vi "produceTimingTicks.vi"(8 "error in (no error)":errorcluster, 10 "Channel":refnum<class "Channel.lvclass">, 11 "PlayFile in":refnum<class "PlayFile.lvclass">) -> (0 "error out":errorcluster, 2 "timingTick":refnum<class "ScriptEventList.lvclass">, 3 "PlayFile out":refnum<class "PlayFile.lvclass">)   [LabVIEW 2011, in "Tools.lvlib" / "Scripting.lvlib" / "PlayFile.lvclass"]
uses:
  PlayFile.lvclass
  DatabaseHelpers/Database Objects/Channel/Channel.lvclass
  ScriptEventList/ScriptEventList.lvclass
  ScriptEvent.lvclass
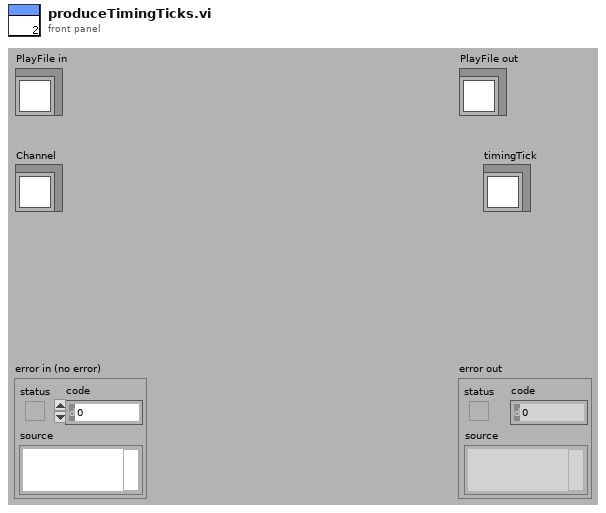
[diagram p1: front panel]
types:
  T1 = enum16{"changeValue", "pulse", "clock", "rampUp", "rampDown", "singleTone", "singleToneRamp", "playFile", "rf", "rfRamp"}
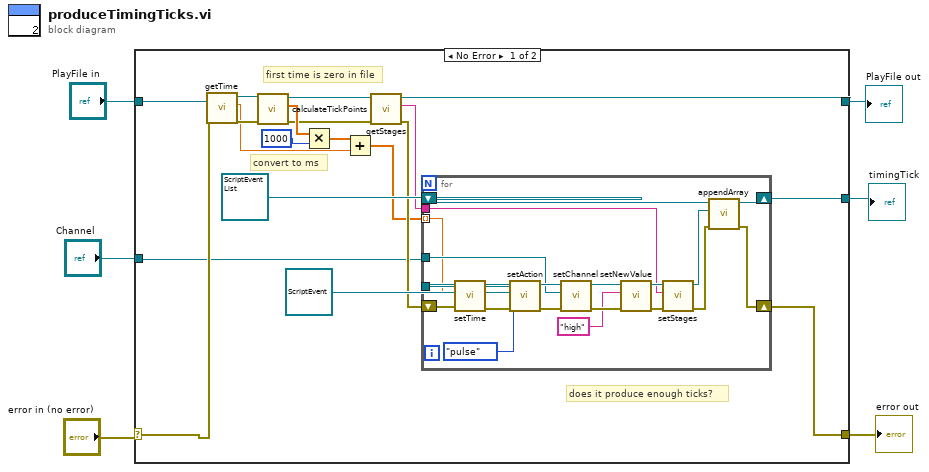
[diagram p0: block diagram]
diagram:
  n1 = case shown="No Error" "error in (no error)" {
    selector: "error in (no error)" -> [w19 w46]
    tunnel: [w20 w47] -> w5
    tunnel: "PlayFile in" -> [w21 w47]
    tunnel: [w7 w46] -> w3
    tunnel: "Channel" -> [w18 _]
    tunnel: [w8 _] -> w1
    frame No Error {
      # "convert to ms"
      # "first time is zero in file"
      # "does it produce enough ticks?"
      n2 = call "getTime.vi"("error in (no error)"=w19, "ScriptEvent.lvclass in"=w21) -> ("error out"=w16:errorcluster, "time"=w15:dbl, "ScriptEvent.lvclass out"=w17:refnum<class "PlayFile.lvclass">)  [unwired: 7 in]
      n3 = call "calculateTickPoints.vi"("error in (no error)"=w16, "PlayFile in"=w17) -> ("error out"=w9:errorcluster, "TimeArray"=w13:dbl[], "PlayFile out"=w10:refnum<class "PlayFile.lvclass">)  [unwired: 7 in]
      n4 = Multiply(x=w13, y=1000) -> (x*y=w14:dbl[])
      n5 = Add(x=w14, y=w15) -> (x+y=w11:dbl[])
      n6 = call "getStages.vi"("error in (no error)"=w9, "ScriptEvent.lvclass in"=w10) -> ("error out"=w23:errorcluster, "Stage"=w22:string, "ScriptEvent.lvclass out"=w20:refnum<class "PlayFile.lvclass">)  [unwired: 7 in]
      n7 = for {
        tunnel: w11 -> [w26] mode=indexing
        tunnel: refnum<class "ScriptEvent.lvclass"> refnum ("Tools.lvlib:Scripting.lvlib:ScriptEvent.lvclass") -> [w45]
        tunnel: w18 -> [w39]
        shift-right: [w33] -> w7
        shift-left: w23 -> [w44]
        shift-right: [w35] -> w8
        shift-left: refnum<class "ScriptEventList.lvclass"> refnum ("Tools.lvlib:Scripting.lvlib:ScriptEventList.lvclass") -> [w34]
        tunnel: w22 -> [w28]
        n8 = call "setTime.vi"("error in (no error)"=w44, "time"=w26, "ScriptEvent.lvclass in"=w45) -> ("error out"=w42:errorcluster, "ScriptEvent.lvclass out"=w43:refnum<class "ScriptEvent.lvclass">)  [unwired: 7 in]
        n9 = call "setAction.vi"("error in (no error)"=w42, "action"=T1."pulse", "ScriptEvent.lvclass in"=w43) -> ("error out"=w40:errorcluster, "ScriptEvent.lvclass out"=w41:refnum<class "ScriptEvent.lvclass">)  [unwired: 7 in]
        n10 = call-dynamic "setChannel.vi"("error in (no error)"=w40, "Channel.lvclass"=w39, "ScriptEvent.lvclass in"=w41) -> ("error out"=w37:errorcluster, "ScriptEvent.lvclass out"=w38:refnum<class "ScriptEvent.lvclass">)  [unwired: 7 in]
        n11 = call "setNewValue.vi"("error in (no error)"=w37, "newValue"="high", "ScriptEvent.lvclass in"=w38) -> ("error out"=w31:errorcluster, "ScriptEvent.lvclass out"=w32:refnum<class "ScriptEvent.lvclass">)  [unwired: 7 in]
        n12 = call-dynamic "setStages.vi"("error in (no error)"=w31, "Stage"=w28, "ScriptEvent.lvclass in"=w32) -> ("error out"=w30:errorcluster, "ScriptEvent.lvclass out"=w29:refnum<class "ScriptEvent.lvclass">)  [unwired: 7 in]
        n13 = call "appendArray.vi"("error in (no error)"=w30, "ScriptEvent"=w29, "ScriptEventList in"=w34) -> ("error out"=w33:errorcluster, "ScriptEventList out"=w35:refnum<class "ScriptEventList.lvclass">)  [unwired: 6 in, 1 out]
      }
    }
    frame Error {
    }
  }
  "error out" <- w3
  "PlayFile out" <- w5
  "timingTick" <- w1
